vi "read_data_kn.vi"(8 "error in (no error)":errorcluster, 11 "KNeighbors in":refnum<class "KNeighbors.lvclass">) -> (0 "error out":errorcluster, 2 "data+":T1={"n_neighbors"=0.0, "mode"="connectivity", "return_distance"=TRUE}, 3 "KNeighbors out":refnum<class "KNeighbors.lvclass">)   [LabVIEW 2020, in "KNeighbors.lvclass"]
uses:
  KNeighbors.lvclass
  Controls/kneighbors_data.ctl
  KNeighbors.lvclass/KNeighbors.ctl
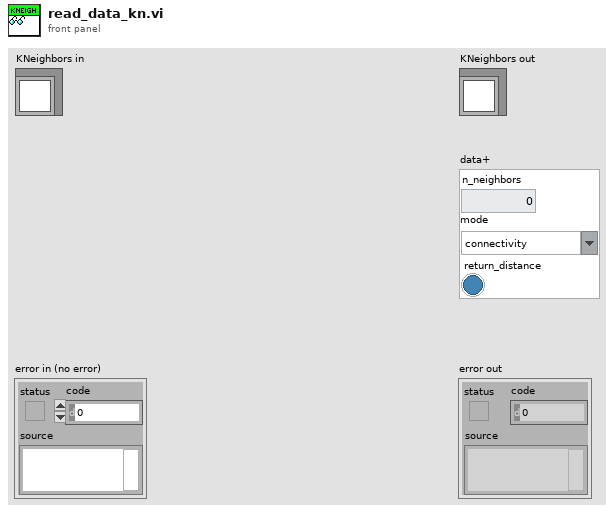
[diagram p1: front panel]
types:
  T1 = typedef "kneighbors_data.ctl" = cluster{"n_neighbors":dbl, "mode":string, "return_distance":bool}
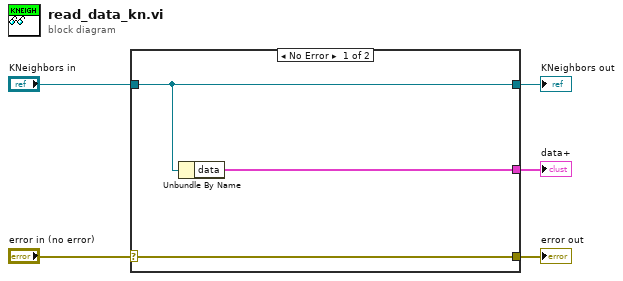
[diagram p0: block diagram]
diagram:
  n1 = case shown="No Error" "error in (no error)" {
    selector: "error in (no error)" -> [w8 w9]
    tunnel: [w8 w9] -> w4
    tunnel: [w7 w10] -> w2
    tunnel: "KNeighbors in" -> [w7 w10]
    tunnel: [w6 _] -> w1
    frame No Error {
      n2 = Unbundle By Name(w7) -> ("data"=w6:T1)
    }
    frame Error {
    }
  }
  "error out" <- w4
  "KNeighbors out" <- w2
  "data+" <- w1
